vi "Load Config.vi"(8 "error in (no error)":errorcluster, 11 "Historian Module in":refnum<class "Historian Module.lvclass">) -> (0 "error out":errorcluster, 3 "Historian Module out":refnum<class "Historian Module.lvclass">)   [LabVIEW 2020, in "VolatusHistorian.lvlib" / "Historian Module.lvclass"]
uses:
  Historian Module.lvclass
  C:/dev/lv20CE/relink/lv-volatus/Volatus/Module/Module.lvclass
  Historian Role.ctl
  Volatus/Module/Module.lvclass/Module.ctl
  VolatusConfig/VolatusConfigElement/VolatusConfigElement.lvclass/VolatusConfigElement.ctl
  Historian Module.lvclass/Historian Module.ctl
  Volatus/Module/Config.vi
  VolatusConfig/VolatusConfigElement/Element.vi
  VolatusConfig/Task/Task Config.lvclass
  C:/dev/lv20CE/relink/lv-volatus/VolatusConfig/VolatusConfigElement/VolatusConfigElement.lvclass
  Volatus/Module/Module.lvclass
  VolatusConfig/VolatusConfigElement/VolatusConfigElement.lvclass
  lv-cdm/CDM-Config/Config Element/Config Element.lvclass
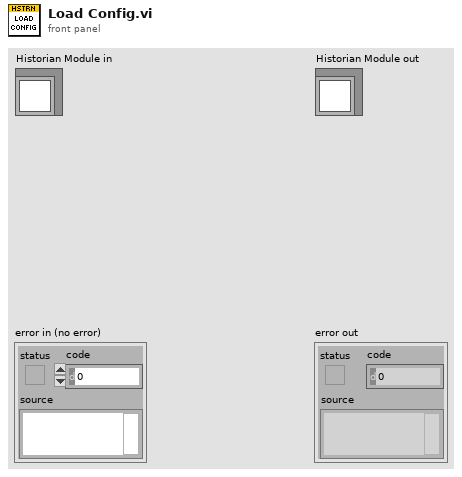
[diagram p1: front panel]
types:
  T1 = typedef "VolatusHistorian.lvlib/Historian Module.lvclass/Historian Role.ctl" = enum16{"Primary", "Local"}
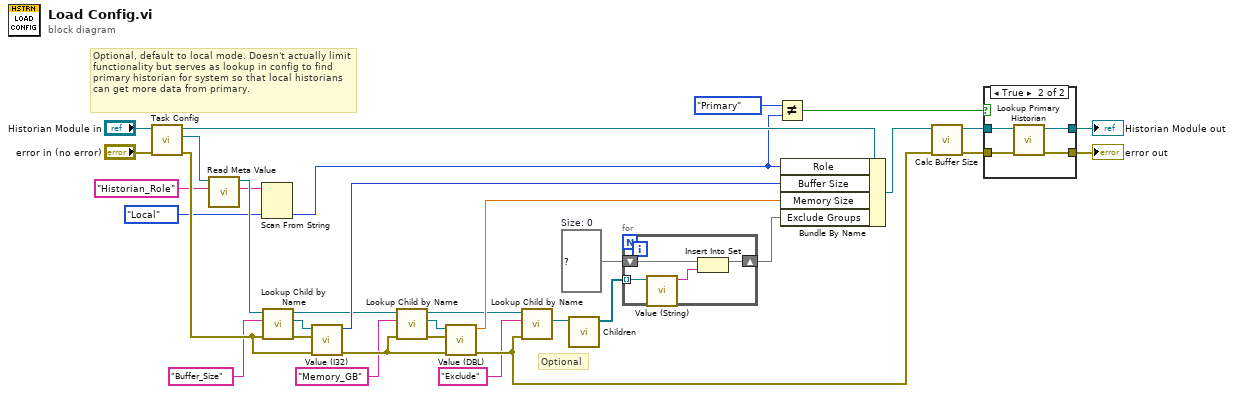
[diagram p0: block diagram]
diagram:
  w22 = set{string} {}  # Size: 0
  # "Optional, default to local mode. Doesn't actually limit functionality but serves as lookup in config to find primary historian for system so that local historians can get more data from primary."
  # "Optional"
  n1 = call "Task Config.vi"("error in (no error)"="error in (no error)", "Module in"="Historian Module in") -> ("error out"=w32:errorcluster, "Task Config"=w20:refnum<class "Task Config.lvclass">, "Module out"=w29:refnum<class "Historian Module.lvclass">)  [unwired: 7 in]
  n2 = call "Read Meta Value.vi"("Meta Name"="Historian_Role", "VolatusConfigElement in"=w20) -> ("Meta Value"=w17:string, "VolatusConfigElement out"=w18:refnum<class "Task Config.lvclass">)  [unwired: 7 in, 1 out]
  n3 = Scan From String(input string=w17, default 1=Historian_Role."Local" ("Historian Role")) -> (output 1=w14:T1)  [unwired: 3 in, 3 out]
  n4 = call "Lookup Child by Name.vi"("error in (no error)"=w32, "Child Name"="Buffer_Size", "VolatusConfigElement in"=w18) -> ("error out"=w26:errorcluster, "Child"=w27:refnum<class "Config Element.lvclass">, "VolatusConfigElement out"=w5:refnum<class "Task Config.lvclass">)  [unwired: 5 in, 1 out]
  n5 = call "Value (I32).vi"("error in (no error)"=w26, "Config Element in"=w27) -> ("I32 Value"=w25:i32)  [unwired: 8 in, 1 out]
  n6 = call "Lookup Child by Name.vi"("error in (no error)"=w32, "Child Name"="Memory_GB", "VolatusConfigElement in"=w5) -> ("error out"=w9:errorcluster, "Child"=w8:refnum<class "Config Element.lvclass">, "VolatusConfigElement out"=w1:refnum<class "Task Config.lvclass">)  [unwired: 5 in, 1 out]
  n7 = call "Value (DBL).vi"("error in (no error)"=w9, "Config Element in"=w8) -> ("DBL Value"=w6:dbl)  [unwired: 8 in, 1 out]
  n8 = call "Lookup Child by Name.vi"("error in (no error)"=w32, "Child Name"="Exclude", "VolatusConfigElement in"=w1) -> ("Child"=w24:refnum<class "Config Element.lvclass">)  [unwired: 5 in, 3 out]
  n9 = call "Children.vi"("Config Element in"=w24) -> ("Elements"=w23:refnum<class "Config Element.lvclass">[])  [unwired: 9 in, 1 out]
  n10 = for {
    tunnel: w23 -> [w36] mode=indexing
    shift-right: [w33] -> w21
    shift-left: w22 -> [w35]
    n11 = call "Value (String).vi"("Config Element in"=w36) -> ("String Value"=w34:string)  [unwired: 9 in, 1 out]
    n12 = Insert Into Set(10:w34, 11:w35) -> (3:w33:set{string})  [unwired: 1 out]
  }
  n13 = Not Equal?(x=Historian_Role."Primary", y=w14) -> (x != y?=w11:bool)
  n14 = Bundle By Name(cluster=w29, "Role"=w14, "Buffer Size"=w25, "Memory Size"=w6, "Exclude Groups"=w21) -> (w4:refnum<class "Historian Module.lvclass">)
  n15 = call "Calc Buffer Size.vi"("error in (no error)"=w32, "Historian Module in"=w4) -> ("error out"=w2:errorcluster, "Historian Module out"=w3:refnum<class "Historian Module.lvclass">)  [unwired: 8 in]
  n16 = case shown="True" w11 {
    tunnel: w3 -> [w38 w42]
    tunnel: [w38 w41] -> w13
    tunnel: w2 -> [w37 w40]
    tunnel: [w37 w39] -> w12
    frame False {
    }
    frame True {
      n17 = call "Lookup Primary Historian.vi"("error in (no error)"=w40, "Historian Module in"=w42) -> ("error out"=w39:errorcluster, "Historian Module out"=w41:refnum<class "Historian Module.lvclass">)  [unwired: 8 in]
    }
  }
  "error out" <- w12
  "Historian Module out" <- w13
